vi "traceSnap.vi"() -> ()   [LabVIEW 2012]
uses:
  <vilib>/userdefined/High Color/IMAQdx.ctl
  <vilib>/vision/driver/NI_Vision_Acquisition_Software.lvlib
panel:
  out "Image Out":T1(plugin-control)
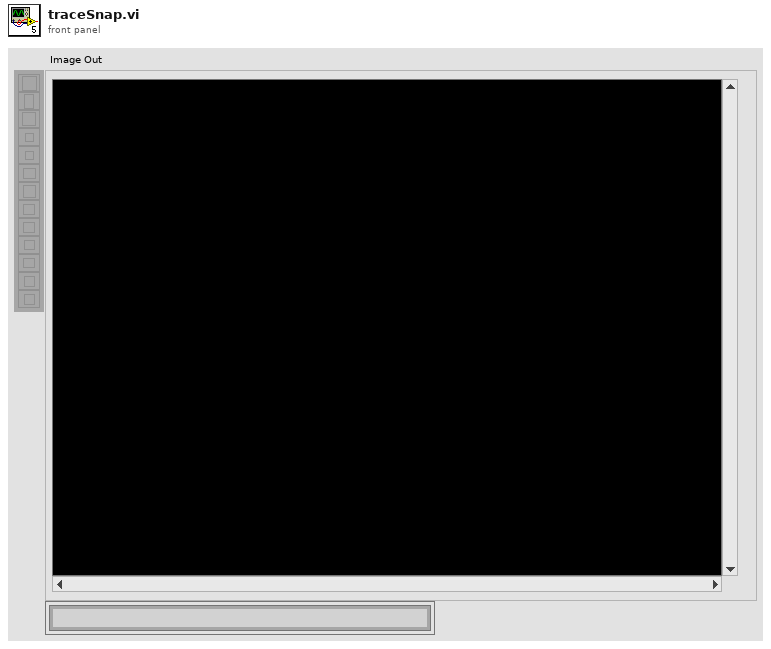
[diagram p1: front panel]
types:
  T1 = typedef "IMAQ Image.ctl" = refnum<image>
  T2 = typedef "Image Type" = u32
  T3 = typedef "IMAQdx.ctl" = refnum<k21>
  T4 = cluster{"Position":cluster{"x":sgl, "y":sgl}, "Angle":sgl, "Scale":sgl, "Score":sgl, "Bounding Box":cluster{"x":sgl, "y":sgl}[]}[]
  T5 = cluster{"Matches (Pattern Matching 1)[0]":cluster{"Position":cluster{"x":sgl, "y":sgl}, "Angle":sgl, "Scale":sgl, "Score":sgl, "Bounding Box":cluster{"x":sgl, "y":sgl}[]}, "Matches (Pattern Matching 1)[1]":cluster{"Position":cluster{"x":sgl, "y":sgl}, "Angle":sgl, "Scale":sgl, "Score":sgl, "Bounding Box":cluster{"x":sgl, "y":sgl}[]}, "Matches (Pattern Matching 1)[2]":cluster{"Position":cluster{"x":sgl, "y":sgl}, "Angle":sgl, "Scale":sgl, "Score":sgl, "Bounding Box":cluster{"x":sgl, "y":sgl}[]}, "Matches (Pattern Matching 1)[3]":cluster{"Position":cluster{"x":sgl, "y":sgl}, "Angle":sgl, "Scale":sgl, "Score":sgl, "Bounding Box":cluster{"x":sgl, "y":sgl}[]}}
  T6 = cluster{"Bounding Box[0]":cluster{"x":sgl, "y":sgl}, "Bounding Box[1]":cluster{"x":sgl, "y":sgl}, "Bounding Box[2]":cluster{"x":sgl, "y":sgl}, "Bounding Box[3]":cluster{"x":sgl, "y":sgl}, "Bounding Box[4]":cluster{"x":sgl, "y":sgl}, "Bounding Box[5]":cluster{"x":sgl, "y":sgl}, "Bounding Box[6]":cluster{"x":sgl, "y":sgl}, "Bounding Box[7]":cluster{"x":sgl, "y":sgl}, "Bounding Box[8]":cluster{"x":sgl, "y":sgl}}
  T7 = cluster{"[0]":sgl, "[1]":sgl, "[2]":sgl, "[3]":sgl}
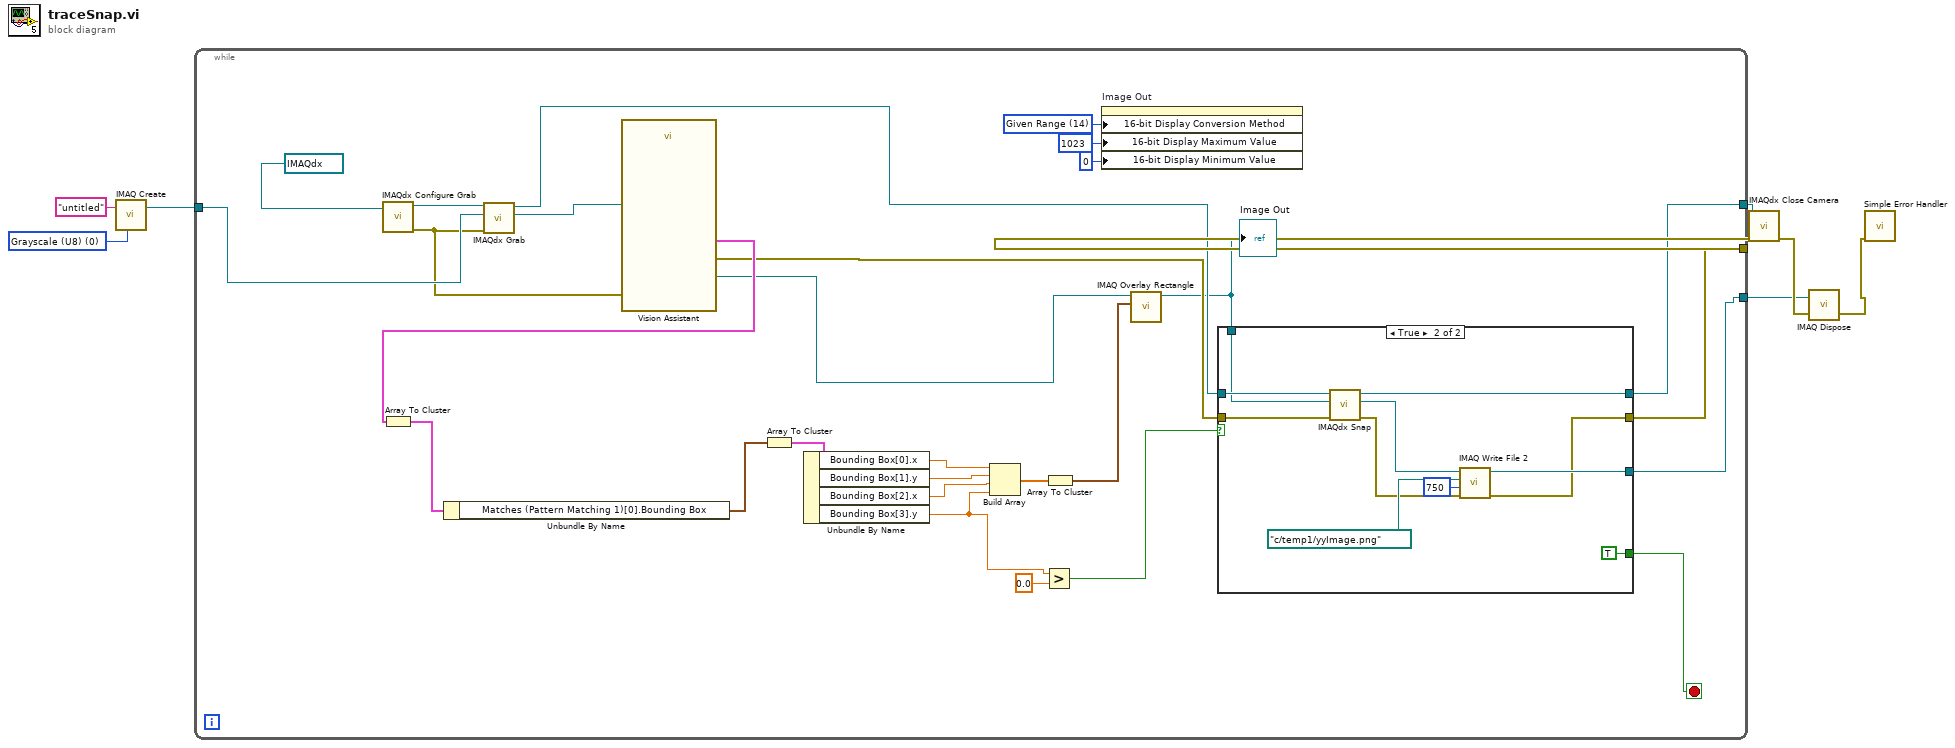
[diagram p0: block diagram]
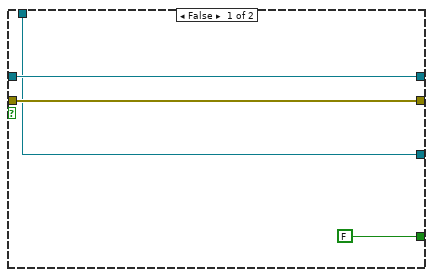
[diagram p2: hidden frame]
diagram:
  w7 = T2 0 items=["Grayscale (U8)", "Grayscale (I16)", "Grayscale (SGL)", "Complex (CSG)", "RGB (U32)", "HSL (U32)", "RGB (U64)", "Grayscale (U16)"] ("Image Type")
  n1 = call "IMAQ Create"("Image Name"="untitled", "Image Type"=w7) -> ("New Image"=w6:T1)  [unwired: 3 in, 1 out]
  n2 = while {
    tunnel: w6 -> [w35]
    tunnel: [w18] -> w3
    tunnel: [w16] -> w2
    tunnel: [w14] -> w1
    stop <- w13 stop-if-true
    w11 = u32 14 items=["Default"=10, "Most Significant Bits"=11, "Full Dynamic"=12, "Downshift"=13, "Given Range"=14, "90% Dynamic"=15, "Given Percent Range"=16] ("16-bit Display Mapping:Conversion Method")
    n3 = call <vilib>:"IMAQdx Configure Grab.vi"("Session In"=T3 "cam0") -> ("error out"=w12:errorcluster, "Session Out"=w36:T3)  [unwired: 9 in]
    n4 = call <vilib>:"IMAQdx Grab.vi"("error in"=w12, "Image In"=w35, "Session In"=w36) -> ("Image Out"=w34:T1, "Session Out"=w19:T3)  [unwired: 5 in, 2 out]
    n5 = call "Vision Assistant"("Image In"=w34, "error in"=w12) -> ("Image Out"=w24:T1, "Matches (Pattern Matching 1)"=w25:T4, "error out"=w17:errorcluster)  [unwired: 23 in]
    n6 = Array To Cluster(array=w25) -> (cluster=w33:T5)
    n7 = Unbundle By Name(w33) -> ("Matches (Pattern Matching 1)[0].Bounding Box"=w32:cluster{"x":sgl, "y":sgl}[])
    n8 = Array To Cluster(array=w32) -> (cluster=w31:T6)
    n9 = Unbundle By Name(w31) -> ("Bounding Box[0].x"=w30:sgl, "Bounding Box[1].y"=w29:sgl, "Bounding Box[2].x"=w28:sgl, "Bounding Box[3].y"=w22:sgl)
    n10 = Build Array(w30, w29, w28, w22) -> (w27:sgl[])
    n11 = Greater?(x=w22, y=sgl 0.0) -> (0:w20:bool)
    n12 = Array To Cluster(array=w27) -> (cluster=w26:T7)
    n13 = property on="Image Out" class="ImageControl"("16-bit Display Conversion Method"=w11, "16-bit Display Maximum Value"=1023 ("16-bit Display Mapping:Maximum Value"), "16-bit Display Minimum Value"=0 ("16-bit Display Mapping:Minimum Value")) -> ()  [unwired: 2 in, 2 out]
    n14 = call "IMAQ Overlay Rectangle"("Rectangle"=w26, "Image"=w24) -> ("Image Out"=w15:T1)  [unwired: 8 in, 1 out]
    "Image Out" <- w15
    n15 = case shown="True" w20 {
      tunnel: w19 -> [w40 w51]
      tunnel: [w40 w50] -> w18
      tunnel: w17 -> [w39 w49]
      tunnel: [w39 w42] -> w16
      tunnel: w15 -> [w38 w48]
      tunnel: [w38 w44] -> w14
      tunnel: [FALSE TRUE] -> w13
      frame False {
      }
      frame True {
        n16 = call <vilib>:"IMAQdx Snap.vi"("error in"=w49, "Image In"=w48, "Session In"=w51) -> ("error out"=w43:errorcluster, "Image Out"=w46:T1, "Session Out"=w50:T3)  [unwired: 6 in]
        n17 = call-poly "IMAQ Write File 2"("error in (no error)"=w43, "Image Quality"=u32 750, "File Path"=path "c:/temp1/yyImage.png", "Image"=w46) -> ("error out"=w42:errorcluster, "Image Out (duplicate)"=w44:T1)  [unwired: 6 in]
      }
    }
  }
  n18 = call <vilib>:"IMAQdx Close Camera.vi"("error in"=w2, "Session In"=w3) -> ("error out"=w5:errorcluster)  [unwired: 9 in]
  n19 = call "IMAQ Dispose"("Image"=w1, "error in (no error)"=w5) -> ("error out"=w4:errorcluster)  [unwired: 1 in, 3 out]
  n20 = call <vilib>:"Simple Error Handler.vi"("error in (no error)"=w4) -> ()  [unwired: 1 in, 8 out]
